vi "Send Data Statistics to Notebook.vi"(6 "Source Data Type (Plot Y Axis)":T1, 7 "Graph Caption":string, 8 "Error In":errorcluster, 9 "Bin":dbl, 10 "Data Statistics":T2, 11 "Plot/Dataset Name":string) -> (0 "Error Out":errorcluster, 1 "Message":string)   [LabVIEW 2021, in "Histogram Window.lvlib"]
uses:
  Histogram Window.lvlib
  Histogram Data Statistics.ctl
  Source Data Type.ctl
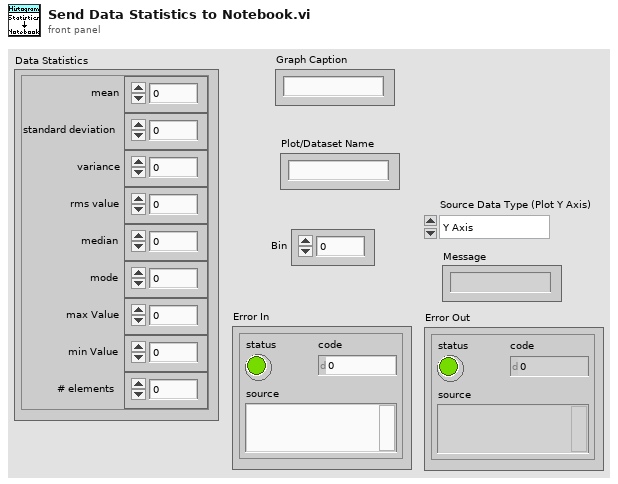
[diagram p1: front panel]
types:
  T1 = typedef "Histogram Window.lvlib/Source Data Type.ctl" = enum16{"Y Axis", "X Axis", "Single Array"}
  T2 = typedef "Histogram Window.lvlib/Histogram Data Statistics.ctl" = cluster{"mean":dbl, "standard deviation":dbl, "variance":dbl, "rms value":dbl, "median":dbl, "mode":dbl, "max Value":dbl, "min Value":dbl, "# elements  ":dbl}
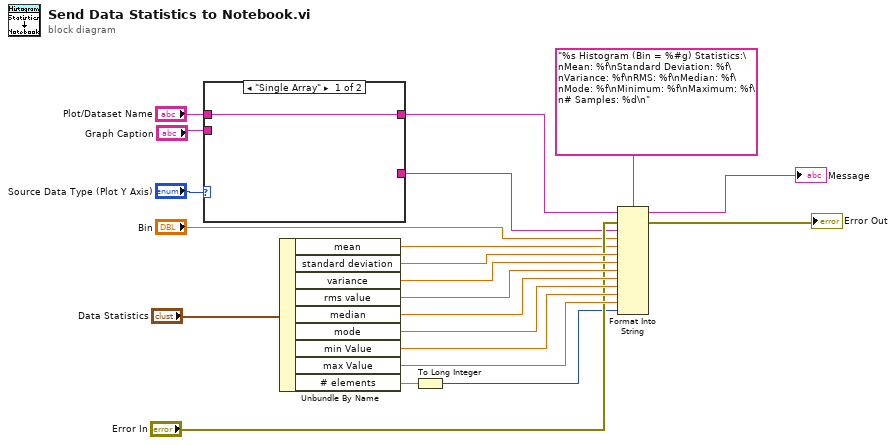
[diagram p0: block diagram]
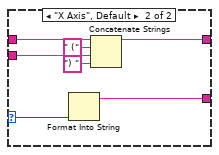
[diagram p2: hidden frame]
diagram:
  n1 = case shown="\"Single Array\"" "Source Data Type (Plot Y Axis)" {
    selector: "Source Data Type (Plot Y Axis)" -> [_ w24]
    tunnel: "Plot/Dataset Name" -> [w22 w29]
    tunnel: "Graph Caption" -> [_ w28]
    tunnel: [w22 w25] -> w3
    tunnel: [_ w23] -> w2
    frame "Single Array" {
    }
    frame "X Axis", Default {
      n2 = Format Into String(w24) -> (resulting string=w23:string)  [unwired: 3 in, 1 out]
      n3 = Concatenate Strings(w29, " (" ("string"), w28, ") " ("string")) -> (w25:string)
    }
  }
  n4 = Unbundle By Name("Data Statistics") -> ("mean"=w5:dbl, "standard deviation"=w18:dbl, "variance"=w17:dbl, "rms value"=w16:dbl, "median"=w15:dbl, "mode"=w14:dbl, "min Value"=w13:dbl, "max Value"=w12:dbl, "# elements"=w11:dbl)
  n5 = To Long Integer(number=w11) -> (32bit integer=w6:i32)
  n6 = Format Into String(format string="%s Histogram (Bin = %#g) Statistics:\nMean: %f\nStandard Deviation: %f\nVariance: %f\nRMS: %f\nMedian: %f\nMode: %f\nMinimum: %f\nMaximum: %f\n# Samples: %d\n", initial string=w3, error in="Error In", w2, "Bin", w5, w18, w17, w16, w15, w14, w13, w12, w6) -> (resulting string=→"Message":string, error out=→"Error Out":errorcluster)
